vi "SV Gen Generate Signal Voltage Waveform.vi"(0 "Signal Generation Settings":T1={"Generation Type"=enum."Single Tone", "Generation Time (s)"=0.1, "Voltage Offset (v)"=0.0, "Single Tone Settings"={"Waveform Type"=enum."Sine Wave", "Frequency (Hz)"=100.0, "Amplitude (V)"=1.0, "Duty Cycle (%)"=50.0}, "Multi Tone Settings"=[]} {"Voltage Offset (v)" format="%#.2p"; "Generation Time (s)" format="%#.2p"; "Multi Tone Settings"."Amplitude (V)" format="%#.2p"; "Multi Tone Settings"."Frequency (Hz)" format="%#.2p"; "Single Tone Settings"."Duty Cycle (%)" format="%#.2p"; "Single Tone Settings"."Amplitude (V)" format="%#.2p"; "Single Tone Settings"."Frequency (Hz)" format="%#.2p"}, 5 "Timing Settings":T6={"Sample Clock Source"="OnboardClock", "Sample Rate (Hz)"=100000.0} {"Sample Rate (Hz)" format="%#.2p"}, 11 "error in":errorcluster) -> (4 "Generated Voltage Waveforms":waveform(dbl)(graph), 15 "error out":errorcluster)   [LabVIEW 2021, in "DAQ_Signal Voltage Generation.lvlib"]
doc: "<B>Generate Signal Voltage Waveform</B> will generate a voltage waveform of either single tone or multi tone type. The waveform are generated with the given Frequency(Hz), Amplitude(V) and Duty cycle(%) supplied as input over the given Generation Time(s)."
uses:
  DAQ_Signal Voltage Generation.lvlib
  Typedefs/Timing Settings.ctl
  Typedefs/Signal Generation Settings.ctl
  Typedefs/Generation Types.ctl
  Typedefs/Single Tone Settings.ctl
  Typedefs/Waveform Type.ctl
  Typedefs/Tone Settings.ctl
  <vilib>/measure/NI_MABase.lvlib
  <vilib>/measure/NI_MAPro.lvlib
panel:
  # "Outputs"
  # "Inputs"
  # "Frequency (Hz)"
  # "Amplitude (V)"
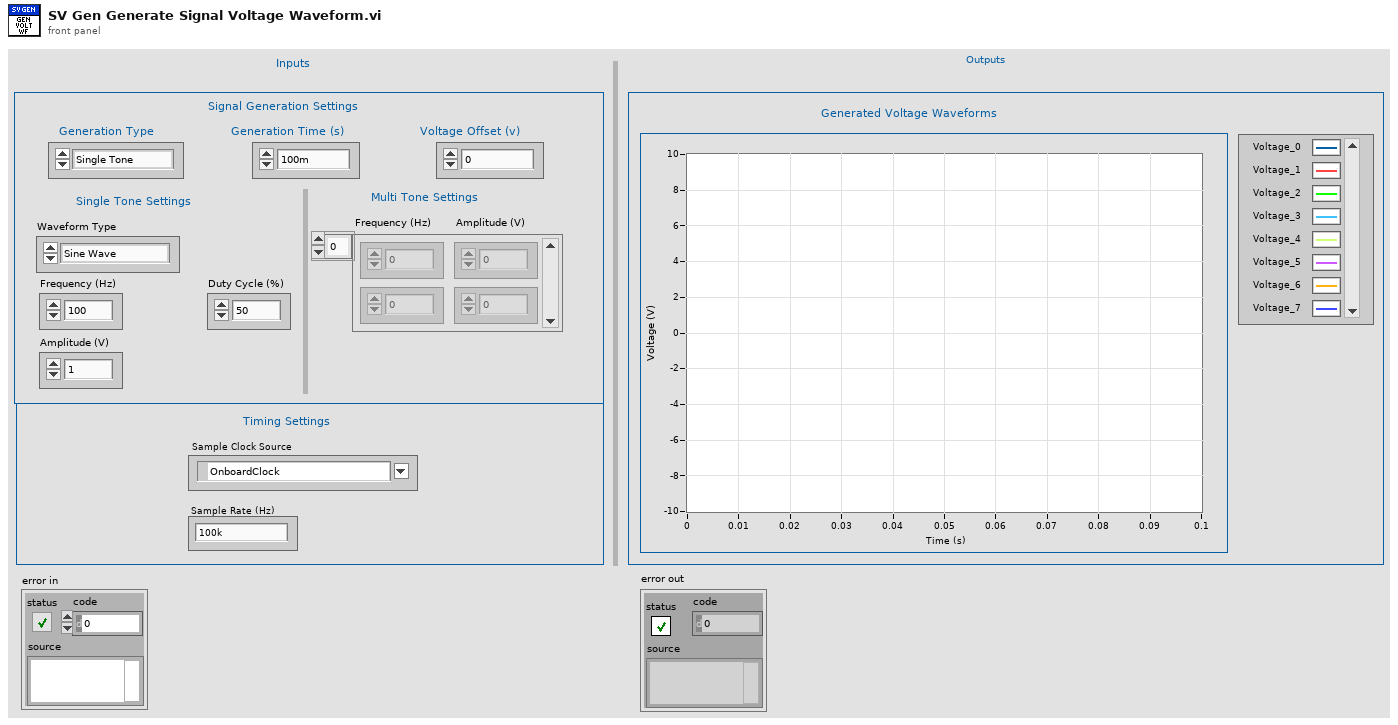
[diagram p1: front panel]
types:
  T1 = typedef "DAQ_Signal Voltage Generation.lvlib/Signal Generation Settings.ctl" = cluster{"Generation Type":T2, "Generation Time (s)":dbl, "Voltage Offset (v)":dbl, "Single Tone Settings":T3, "Multi Tone Settings":T5[]}
  T2 = typedef "DAQ_Signal Voltage Generation.lvlib/Generation Types.ctl" = enum16{"Single Tone", "Multi Tone"}
  T3 = typedef "DAQ_Signal Voltage Generation.lvlib/Single Tone Settings.ctl" = cluster{"Waveform Type":T4, "Frequency (Hz)":dbl, "Amplitude (V)":dbl, "Duty Cycle (%)":dbl}
  T4 = typedef "DAQ_Signal Voltage Generation.lvlib/Waveform Type.ctl" = enum16{"Sine Wave", "Square Wave"}
  T5 = typedef "DAQ_Signal Voltage Generation.lvlib/Tone Settings.ctl" = cluster{"Frequency (Hz)":dbl, "Amplitude (V)":dbl}
  T6 = typedef "DAQ_Signal Voltage Generation.lvlib/Timing Settings.ctl" = cluster{"Sample Clock Source":tag, "Sample Rate (Hz)":dbl}
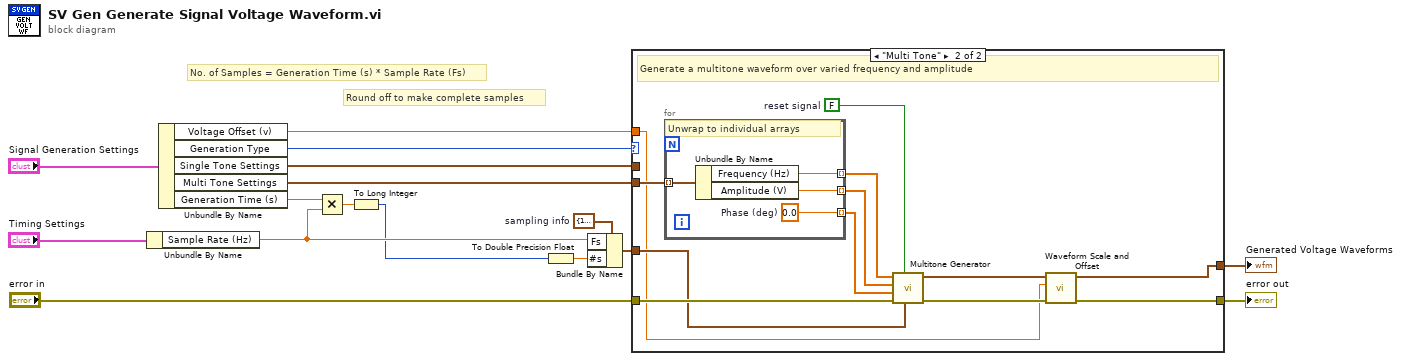
[diagram p0: block diagram]
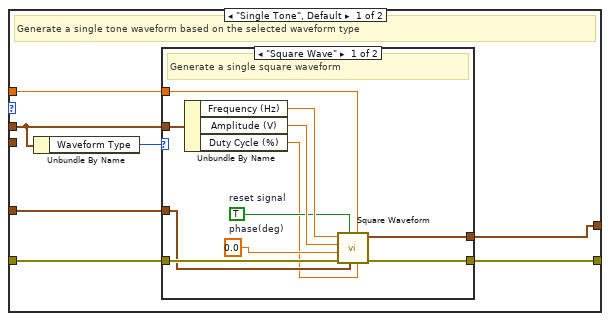
[diagram p2: hidden frame]
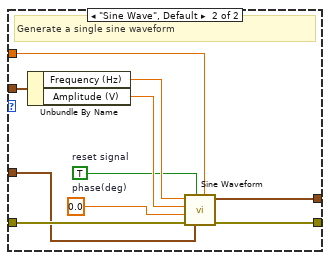
[diagram p3: hidden frame]
diagram:
  w12 = cluster{"Fs":dbl, "#s":dbl} {"Fs"=1000.0, "#s"=1000.0}  # sampling info
  # "Round off to make complete samples"
  # "No. of Samples = Generation Time (s) * Sample Rate (Fs)"
  n1 = Unbundle By Name("Timing Settings") -> ("Sample Rate (Hz)"=w4:dbl)
  n2 = Unbundle By Name("Signal Generation Settings") -> ("Voltage Offset (v)"=w1:dbl, "Generation Type"=w8:T2, "Single Tone Settings"=w7:T3, "Multi Tone Settings"=w6:T5[], "Generation Time (s)"=w5:dbl)
  n3 = Multiply(x=w5, y=w4) -> (x*y=w3:dbl)
  n4 = To Long Integer(number=w3) -> (32bit integer=w2:i32)
  n5 = To Double Precision Float(number=w2) -> (double precision float=w13:dbl)
  n6 = Bundle By Name(cluster=w12, "Fs"=w4, "#s"=w13) -> (w10:cluster{"Fs":dbl, "#s":dbl})
  n7 = case shown="\"Multi Tone\"" w8 {
    tunnel: "error in" -> [w22 w56]
    tunnel: [w21 w48] -> w15
    tunnel: [w20 w45] -> w14
    tunnel: w10 -> [w19 w55]
    tunnel: w7 -> [w18 _]
    tunnel: w6 -> [_ w54]
    tunnel: w1 -> [w17 w46]
    frame "Single Tone", Default {
      # "Generate a single tone waveform based on the selected waveform type"
      n8 = Unbundle By Name(w18) -> ("Waveform Type"=w23:T4)
      n9 = case shown="\"Square Wave\"" w23 {
        tunnel: w22 -> [w34 w44]
        tunnel: w18 -> [w32 w42]
        tunnel: w19 -> [w33 w43]
        tunnel: [w26 w37] -> w20
        tunnel: [w25 w36] -> w21
        tunnel: w17 -> [w24 w35]
        frame "Square Wave" {
          w28 = TRUE  # reset signal
          w29 = 0.0  # phase(deg)
          # "Generate a single square waveform"
          n10 = Unbundle By Name(w32) -> ("Frequency (Hz)"=w31:dbl, "Amplitude (V)"=w30:dbl, "Duty Cycle (%)"=w27:dbl)
          n11 = call <vilib>:"Square Waveform.vi"("duty cycle (%)"=w27, "offset"=w24, "sampling info"=w33, "reset signal"=w28, "error in (no error)"=w34, "phase"=w29, "amplitude"=w30, "frequency"=w31) -> ("error out"=w25:errorcluster, "signal out"=w26:waveform(dbl))  [unwired: 2 in]
        }
        frame "Sine Wave", Default {
          w38 = TRUE  # reset signal
          w39 = 0.0  # phase(deg)
          # "Generate a single sine waveform"
          n12 = Unbundle By Name(w42) -> ("Frequency (Hz)"=w41:dbl, "Amplitude (V)"=w40:dbl)
          n13 = call <vilib>:"Sine Waveform.vi"("offset"=w35, "sampling info"=w43, "reset signal"=w38, "error in (no error)"=w44, "phase"=w39, "amplitude"=w40, "frequency"=w41) -> ("error out"=w36:errorcluster, "signal out"=w37:waveform(dbl))  [unwired: 3 in]
        }
      }
    }
    frame "Multi Tone" {
      w50 = FALSE  # reset signal
      # "Generate a multitone waveform over varied frequency and amplitude"
      n14 = for {
        tunnel: w54 -> [w60] mode=indexing
        tunnel: [w59] -> w53 mode=indexing
        tunnel: [w58] -> w52 mode=indexing
        tunnel: [w57] -> w51 mode=indexing
        w57 = 0.0  # Phase (deg)
        # "Unwrap to individual arrays"
        n15 = Unbundle By Name(w60) -> ("Frequency (Hz)"=w59:dbl, "Amplitude (V)"=w58:dbl)
      }
      n16 = call <vilib>:"Multitone Generator.vi"("sampling info"=w55, "reset signal"=w50, "error in (no error)"=w56, "tone phases"=w51, "tone amplitudes"=w52, "tone frequencies"=w53) -> ("error out"=w49:errorcluster, "signal out"=w47:waveform(dbl))  [unwired: 2 in, 2 out]
      n17 = call <vilib>:"Waveform Scale and Offset.vi"("error in (no error)"=w49, "offset"=w46, "waveform in"=w47) -> ("error out"=w48:errorcluster, "waveform out"=w45:waveform(dbl))  [unwired: 7 in]
    }
  }
  "error out" <- w15
  "Generated Voltage Waveforms" <- w14
